vi "ErrorHandler.vi"(8 "error in (no error)":errorcluster, 11 "Handler in":refnum<class "Handler.lvclass">) -> (0 "error out":errorcluster, 3 "Handler out":refnum<class "Handler.lvclass">)   [LabVIEW 2022 SP3, in "Error.lvlib" / "Handler.lvclass"]
uses:
  Handler.lvclass
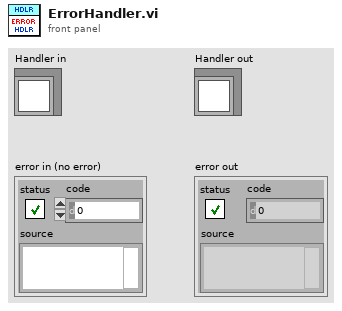
[diagram p1: front panel]
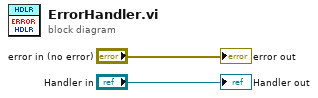
[diagram p0: block diagram]
diagram:
  "error out" <- "error in (no error)"
  "Handler out" <- "Handler in"
